vi "GetParentClassesHiererchy.vi"(8 "error in (no error)":errorcluster, 10 "Classes in memory":refnum<class>[](array[class]), 11 "LabVIEW Object in":refnum<class>) -> (0 "error out":errorcluster, 3 "Class (child,parent)":T1[](array[typedef]))   [LabVIEW 2020, in "BlueSerialization.lvlib" / "BlueSerializer.lvclass"]
uses:
  BlueSerializer.lvclass
  ClassNameObj.ctl
  ClassNameSummary.ctl
  LVOOP is Same or Descendant Class Inline.vi
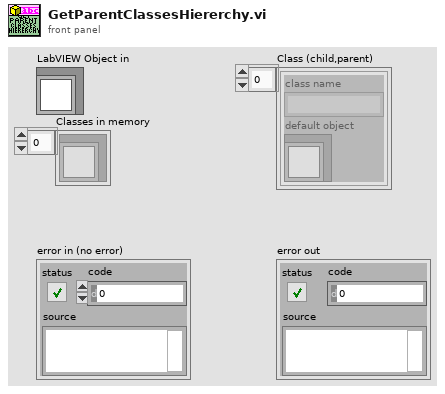
[diagram p1: front panel]
types:
  T1 = typedef "BlueSerialization.lvlib/BlueSerializer.lvclass/ClassNameObj.ctl" = cluster{"class name":string, "default object":refnum<class>}
  T2 = typedef "BlueSerialization.lvlib/BlueSerializer.lvclass/ClassNameSummary.ctl" = enum16{"sibling", "more specific", "less specific", "same"}
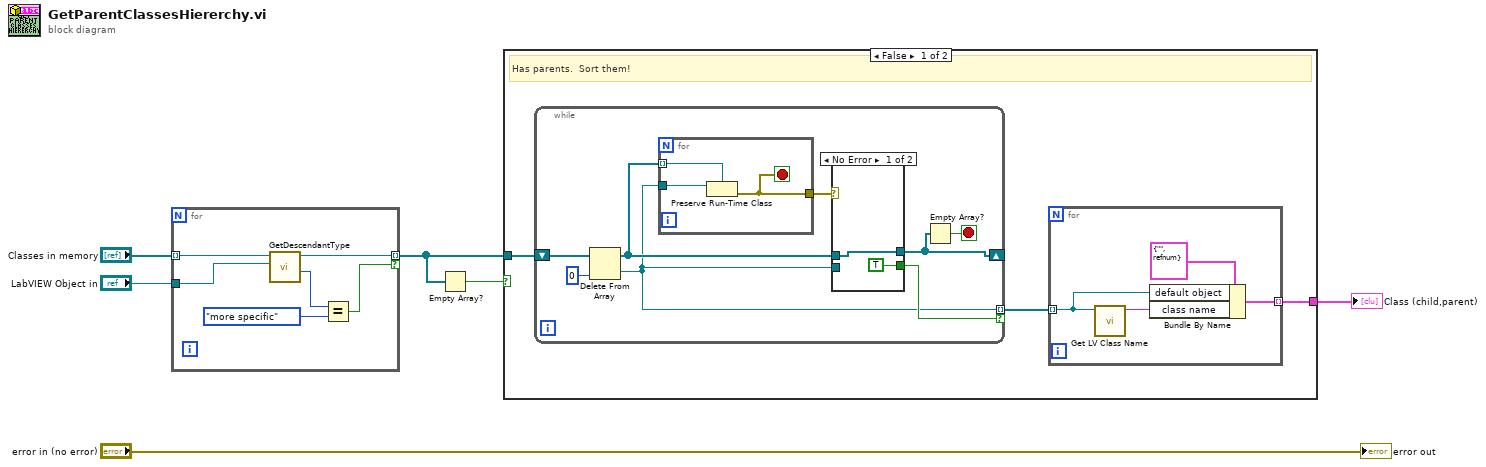
[diagram p0: block diagram]
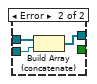
[diagram p2: hidden frame]
diagram:
  n1 = for {
    tunnel: [w10] -> w5 mode=indexing if=w7
    tunnel: "LabVIEW Object in" -> [w9]
    tunnel: "Classes in memory" -> [w11] mode=indexing
    n2 = call "GetDescendantType.vi"("To Object"=w9, "From Object"=w11) -> ("Descent Type"=w8:T2, "From Object (dup)"=w10:refnum<class>)  [unwired: 6 in, 2 out]
    n3 = Equal?(x=w8, y=ClassNameSummary."more specific" ("Descent Type")) -> (x = y?=w7:bool)
  }
  n4 = Empty Array?(array=w5) -> (empty?=w4:bool)
  n5 = case shown="False" w4 {
    tunnel: [w15 _] -> w3
    tunnel: w5 -> [w13 _]
    frame False {
      # "Has parents.  Sort them!"
      n6 = while {
        shift-right: [w16] -> _
        shift-left: w13 -> [w23]
        tunnel: [w17] -> w14 mode=indexing if=w18
        stop <- w20 stop-if-true
        n7 = Delete From Array(array=w23, index=0) -> (deleted portion=w17:refnum<class>, array with subset deleted=w19:refnum<class>[])  [unwired: 1 in]
        n8 = for {
          tunnel: w17 -> [w31]
          tunnel: w19 -> [w30] mode=indexing
          tunnel: [w29] -> w21
          stop <- w29 stop-if-true
          n9 = Preserve Run-Time Class(object in=w31, 2:w30) -> (error out=w29:errorcluster)  [unwired: 1 in, 1 out]
        }
        n10 = case shown="No Error" w21 {
          tunnel: w19 -> [w25 w28]
          tunnel: [w25 w27] -> w16
          tunnel: [TRUE _] -> w18
          tunnel: w17 -> [_ w26]
          frame No Error {
          }
          frame Error {
            n11 = Build Array (concatenate)(w28, w26) -> (w27:refnum<class>[])
          }
        }
        n12 = Empty Array?(array=w16) -> (empty?=w20:bool)
      }
      n13 = for {
        tunnel: w14 -> [w34] mode=indexing
        tunnel: [w32] -> w15 mode=indexing
        n14 = call <vilib>:"Get LV Class Name.vi"("object"=w34) -> ("class name"=w33:string)  [unwired: 9 in, 1 out]
        n15 = Bundle By Name(cluster=T1 {"class name"="", "default object"=refnum} ("Cluster"), "default object"=w34, "class name"=w33) -> (w32:T1)
      }
    }
    frame True {
      # "no parents!  return nothing"
    }
  }
  "Class (child,parent)" <- w3
  "error out" <- "error in (no error)"
